vi "CheckLStat.vi"(8 "error in (no error)":errorcluster, 10 "password":string, 11 "license file path":path) -> (0 "error out":errorcluster, 1 "error code":i32, 2 "license status":T1(ring), 3 "license file handle":i32)   [LabVIEW 2014, in "Raspberry Pi Compatible Compiler for LabVIEW.lvlib"]
uses:
  Raspberry Pi Compatible Compiler for LabVIEW.lvlib
  <resource>/KEYLIB32.dll
panel:
  in  "error code buffer":i32
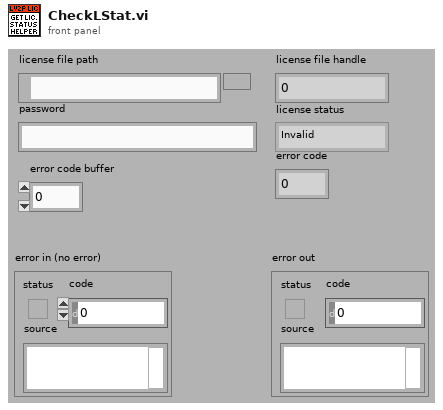
[diagram p1: front panel]
types:
  T1 = enum16{"Invalid", "Expired", "Evaluation", "Activated"}
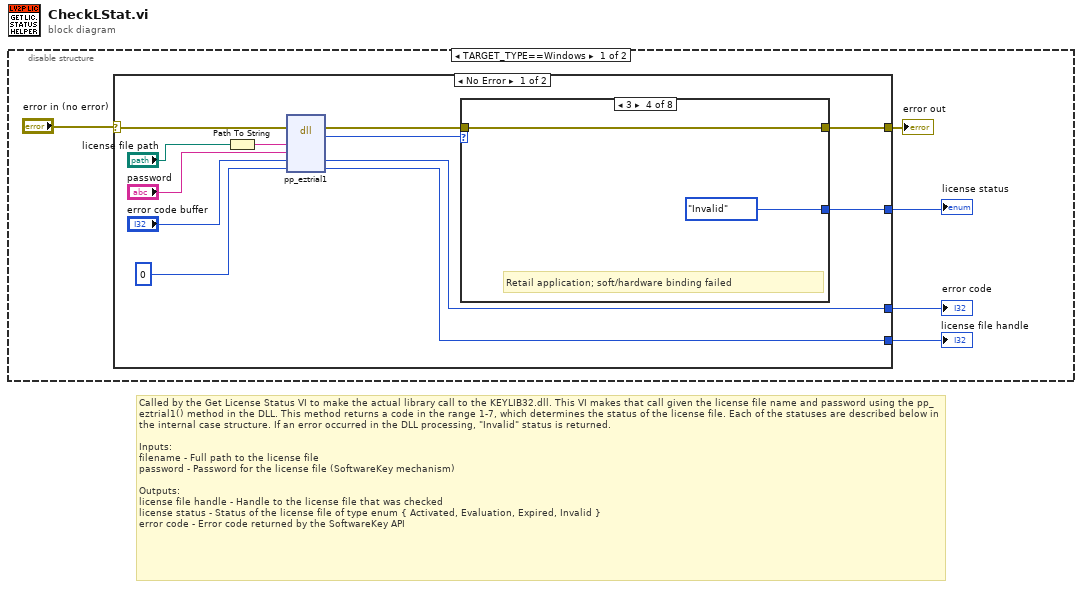
[diagram p0: block diagram]
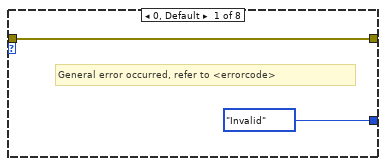
[diagram p2: hidden frame]
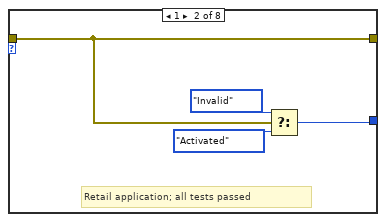
[diagram p3: hidden frame]
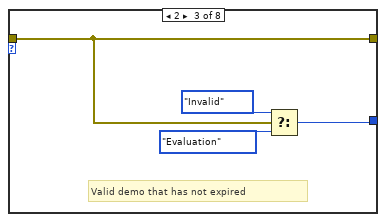
[diagram p4: hidden frame]
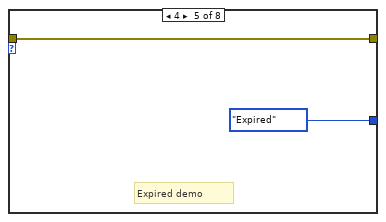
[diagram p5: hidden frame]
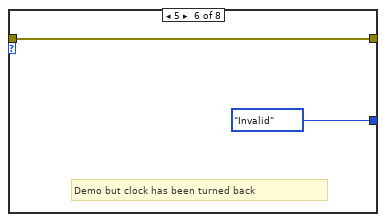
[diagram p6: hidden frame]
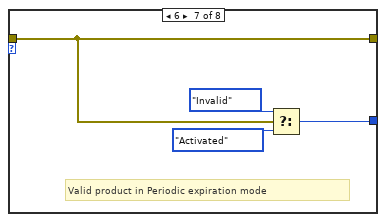
[diagram p7: hidden frame]
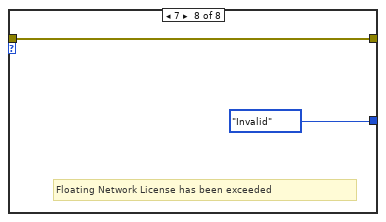
[diagram p8: hidden frame]
diagram:
  # "Called by the Get License Status VI to make the actual library call to the KEYLIB32.dll. This VI makes that call given the license file name and password using the pp_eztrial1() method in the DLL. This method returns a code in the range 1-7, which determines the status of the license file. Each of the statuses are described below in the internal case structure. If an error occurred in the DLL processing, \"Invalid\" status is returned.\n\nInputs:\nfilename - Full path to the license file\npassword - Password for the license file (SoftwareKey mechanism)\n\nOutputs:\nlicense file handle - Handle to the license file that was checked\nlicense status - Status of the license file of type enum { Activated, Evaluation, Expired, Invalid }\nerror code - Error code returned by the SoftwareKey API"
  n1 = disable-structure shown="TARGET_TYPE==Windows" {
    frame condition #0 (active) {
      n2 = case shown="No Error" "error in (no error)" {
        selector: "error in (no error)" -> [w12 w40]
        tunnel: [w14 w40] -> w5
        tunnel: [w11 _] -> w3
        tunnel: [w10 _] -> w2
        tunnel: [w7 _] -> w1
        frame No Error {
          n3 = Path To String(path="license file path") -> (string=w9:string)
          n4 = dll-call lib="C:/Program Files (x86)/National Instruments/LabVIEW 2014/resource/KEYLIB*.dll" fn="pp_eztrial1"(error in=w12, "file"=w9, "password"="password", "error code"="error code buffer", "lfhandle"=0 ("lfhandle (buffer)")) -> (error out=w6:errorcluster, "return type"=w13:i32, "error code"=w10:i32, "lfhandle"=w7:i32)  [unwired: 4 in, 1 out]
          n5 = case shown="3" w13 {
            tunnel: w6 -> [w19 w23 w27 w29 w31 w33 w37 w39]
            tunnel: [w19 w23 w27 w29 w31 w33 w37 w39] -> w14
            tunnel: [T1."Invalid" ("license status 2") w20 w24 T1."Invalid" ("license status 2") T1."Expired" ("license status 2") T1."Invalid" ("license status 2") w34 T1."Invalid" ("license status 2")] -> w11
            frame 0, Default {
              # "General error occurred, refer to <errorcode>"
            }
            frame 1 {
              # "Retail application; all tests passed"
              n6 = Select(t=T1."Invalid" ("license status 2"), s=w23, f=T1."Activated" ("license status 2")) -> (s? t:f=w20:T1)
            }
            frame 2 {
              # "Valid demo that has not expired"
              n7 = Select(t=T1."Invalid" ("license status 2"), s=w27, f=T1."Evaluation" ("license status 2")) -> (s? t:f=w24:T1)
            }
            frame 3 {
              # "Retail application; soft/hardware binding failed"
            }
            frame 4 {
              # "Expired demo"
            }
            frame 5 {
              # "Demo but clock has been turned back"
            }
            frame 6 {
              # "Valid product in Periodic expiration mode"
              n8 = Select(t=T1."Invalid" ("license status 2"), s=w37, f=T1."Activated" ("license status 2")) -> (s? t:f=w34:T1)
            }
            frame 7 {
              # "Floating Network License has been exceeded"
            }
          }
        }
        frame Error {
        }
      }
      "error out" <- w5
      "error code" <- w2
      "license file handle" <- w1
      "license status" <- w3
    }
    frame condition #1 {
    }
  }
